vi "Run.vi"(8 "error in (no error)":errorcluster, 11 "Analog in":refnum<class "Simulated DMM.lvclass">) -> (0 "error out":errorcluster, 3 "Analog out":refnum<class "Simulated DMM.lvclass">)   [LabVIEW 2018, in "Simulated DMM.lvclass"]
uses:
  Simulated DMM.lvclass
  Common Components/Hardware/DMM/DMM.lvclass
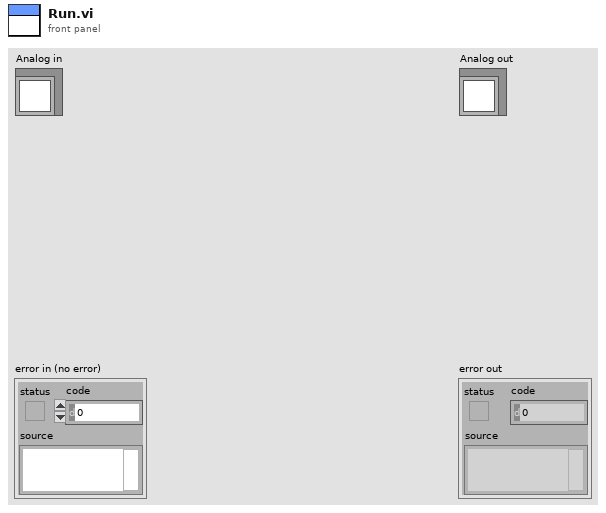
[diagram p1: front panel]
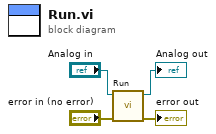
[diagram p0: block diagram]
diagram:
  n1 = call-parent "Run.vi"("error in (no error)"="error in (no error)", "Analog in"="Analog in") -> ("error out"=→"error out":errorcluster, "Analog out"=→"Analog out":refnum<class "Simulated DMM.lvclass">)  [unwired: 8 in]
